vi "Calculate Wing Angle.vi"(2 "Laser D2":dbl, 3 "Laser D1":dbl) -> (0 "Vertical Displacment of wing (mm)":dbl, 1 "Angle of Wing":dbl)   [LabVIEW 2022 SP3]
panel:
  out "D2 Thickness Change":dbl format="%.4f"
  out "D1 Thickness Change":dbl format="%.4f"
  out "Numeric":i32
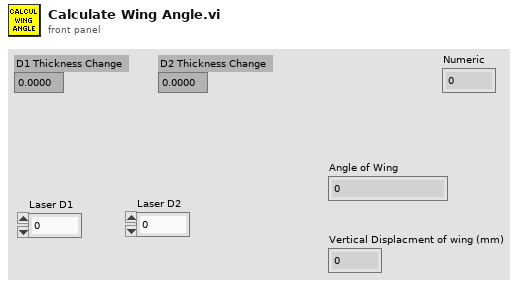
[diagram p1: front panel]
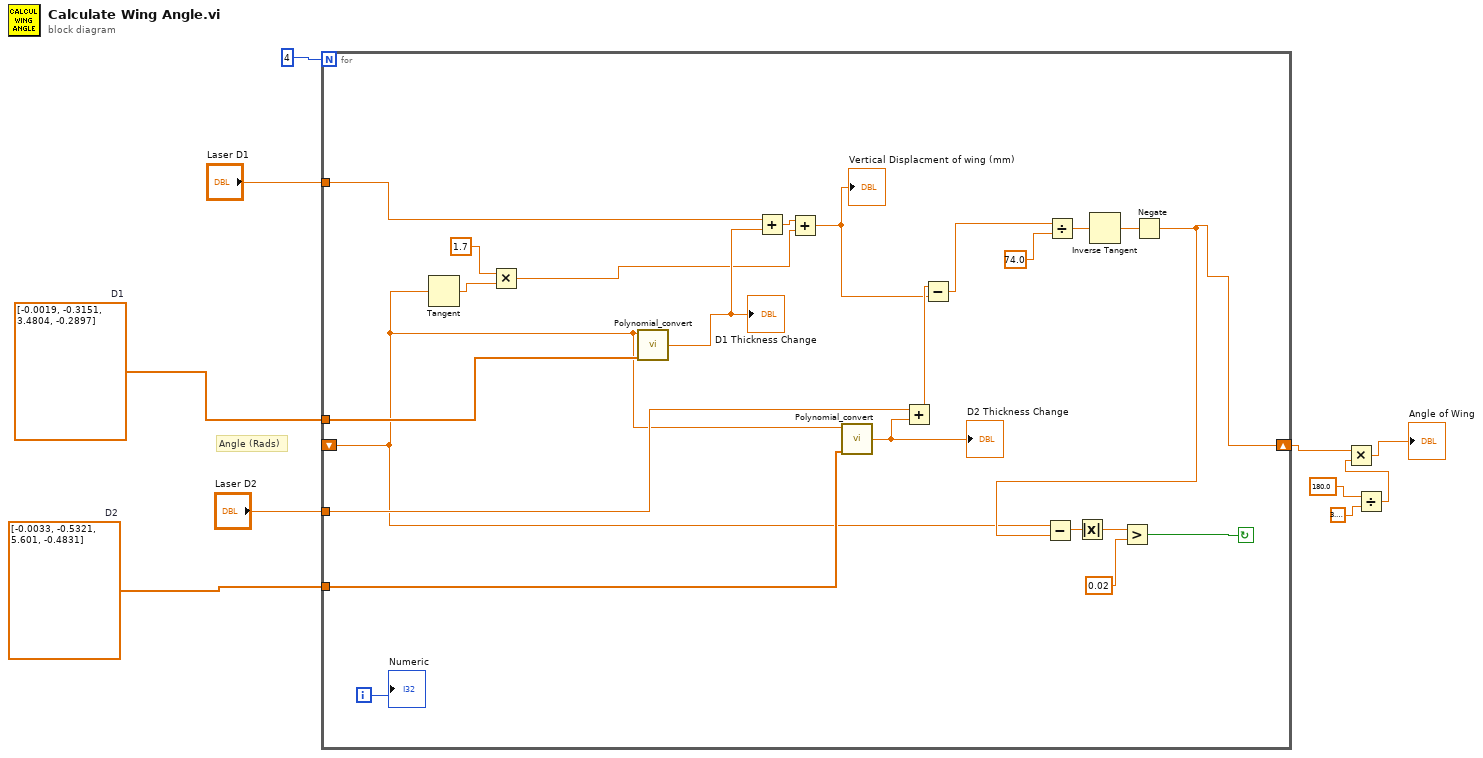
[diagram p0: block diagram]
diagram:
  w3 = dbl[] [-0.0033, -0.5321, 5.601, -0.4831]  # D2
  w4 = dbl[] [-0.0019, -0.3151, 3.4804, -0.2897]  # D1
  # "Angle (Rads)"
  n1 = for {
    N: 4 -> [_]
    shift-right: [w17] -> w7
    shift-left: _ -> [w11]
    tunnel: w4 -> [w30]
    tunnel: w3 -> [w29]
    tunnel: "Laser D1" -> [w28]
    tunnel: "Laser D2" -> [w27]
    i -> [w31]
    stop <- w32 continue-if-true
    n2 = Tangent(1:w11) -> (0:w16:dbl)
    n3 = Multiply(x=1.7, y=w16) -> (x*y=w13:dbl)
    n4 = call "Polynomial_convert.vi"("Calib constants"=w30, "Voltage"=w11) -> ("Eng Values"=w26:dbl)  [unwired: 4 in]
    "D1 Thickness Change" <- w26
    n5 = Add(x=w28, y=w26) -> (x+y=w14:dbl)
    n6 = Add(x=w14, y=w13) -> (x+y=w12:dbl)
    "Vertical Displacment of wing (mm)" <- w12
    n7 = call "Polynomial_convert.vi"("Calib constants"=w29, "Voltage"=w11) -> ("Eng Values"=w25:dbl)  [unwired: 4 in]
    "D2 Thickness Change" <- w25
    n8 = Add(x=w27, y=w25) -> (x+y=w22:dbl)
    n9 = Subtract(x=w22, y=w12) -> (x-y=w21:dbl)
    n10 = Divide(x=w21, y=74.0) -> (x/y=w24:dbl)
    n11 = Inverse Tangent(1:w24) -> (0:w33:dbl)
    n12 = Negate(x=w33) -> (-x=w17:dbl)
    n13 = Subtract(x=w11, y=w17) -> (x-y=w20:dbl)
    n14 = Absolute Value(x=w20) -> (abs(x)=w18:dbl)
    n15 = Greater?(x=w18, y=0.02) -> (0:w32:bool)
    "Numeric" <- w31
  }
  n16 = Divide(x=180.0, y=3.141592653589793) -> (x/y=w6:dbl)
  n17 = Multiply(x=w7, y=w6) -> (x*y=→"Angle of Wing":dbl)
